vi "Run_FFID_Bkgnd.vi"(3 "Simulated Time":timestamp, 4 "Run Now?":bool, 5 "Simulate/Run":T3) -> (0 "Error Messages":string, 2 "Status":T1)   [LabVIEW 2018]
uses:
  Controls/User_Specific_mode.ctl
  Controls/Multirun_Execute_Row_Connector_Pane.ctl
  Gen Trav/Multi_Run_Status.ctl
  Globals/Trav_pos_global.vi
  Globals/Extra_Commands_Global.vi
  Globals/Constants_global.vi
panel:
  in  "User Specific":T2
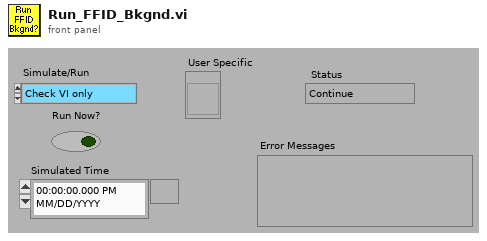
[diagram p1: front panel]
types:
  T1 = typedef "Multi_Run_Status.ctl" = enum16{"Continue", "Continue with Error", "Jump to Next Point", "Jump to Next Row", "Jump To Fall Back", "Terminate Run"}
  T2 = typedef "Multirun_Execute_Row_Connector_Pane.ctl" = refnum<vi>
  T3 = typedef "User_Specific_mode.ctl" = enum16{"Check VI only", "Run VI"}
  T4 = typedef "Traverse_cluster.ctl" = cluster{"Start X":sgl, "Start Y":sgl, "Start Z":sgl, "End X":sgl, "End Y":sgl, "End Z":sgl, "No. of pts.":i32, "Spacing":T5, "Filename":path, "Tunnel Speed":dbl, "Averaging time (min)":dbl, "Extra Commands":string, "Carrier_1 Q (l/min)":dbl, "Carrier_2 Q (l/min)":dbl, "Trace Gas Concentration (%)":dbl, "Specific Arguments":string, "Comments":string, "Row No":i32, "Row Type Selector":T6, "Completion time":string, "Row Duration (mins)":dbl, "No. of Valid pts.":i32, "Meas Setup File":string}
  T5 = typedef "Spacing.ctl" = enum16{"Linear", "Log", "Gauss", "Specified", "N/A"}
  T6 = typedef "Multi_run_mode.ctl" = enum16{"Move Traverse Only", "Set Tunnel Speed Only", "Set Source Only", "Set Measurement Conditions", "Single Measurement", "Vertical Profile", "Lateral Profile", "Longitudinal Profile", "Multi-Axis Profile", "Explore Volume", "Auto Calibrate", "Meas Fast FID Bkgnd", "Check Beam Power", "Scanning Valve Measurement", "Run VI Named:", "Set ADAM Ch", "Wait (minutes)", "Send Message", "Synchronize With:", "Fall Back to this Row", "Turn Off Row Repeating", "Traverse 3D Volume", "Blank Row", "Jump to Fall Back Row"}
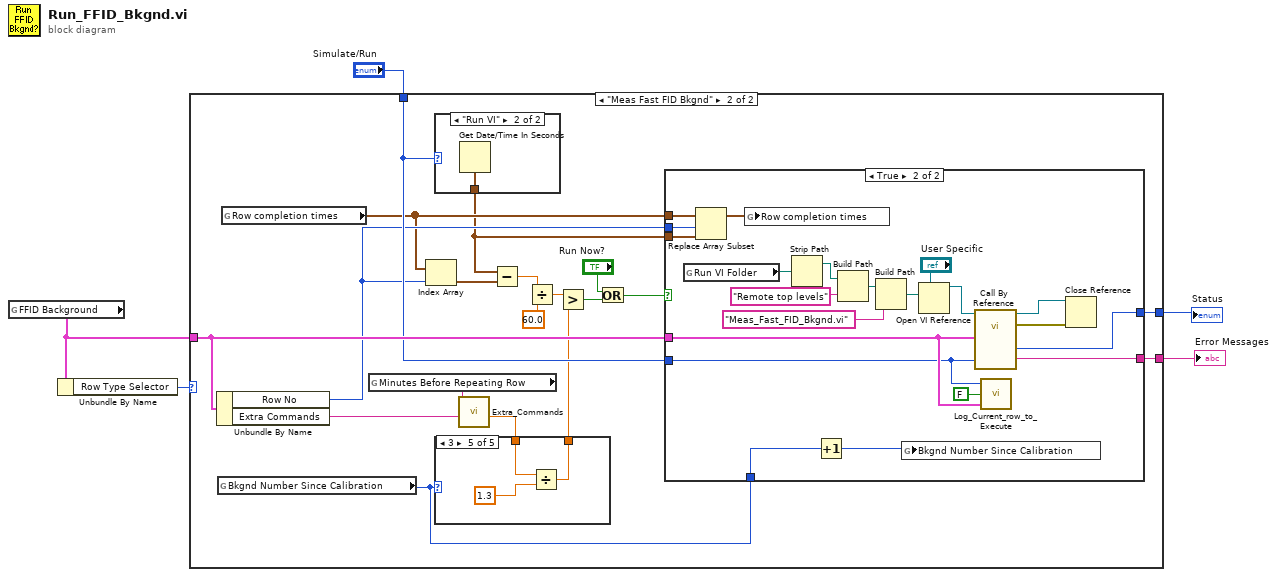
[diagram p0: block diagram]
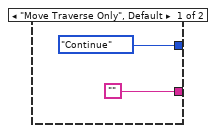
[diagram p2: hidden frame]
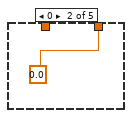
[diagram p4: hidden frame]
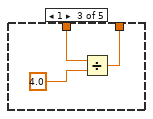
[diagram p5: hidden frame]
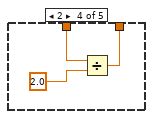
[diagram p6: hidden frame]
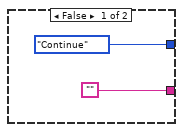
[diagram p7: hidden frame]
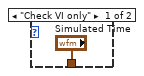
[diagram p8: hidden frame]
diagram:
  n1 = global read "Trav_pos_global.vi" "FFID Background"() -> (w5:T4)
  n2 = Unbundle By Name(w5) -> ("Row Type Selector"=w1:T6)
  n3 = case shown="\"Meas Fast FID Bkgnd\"" w1 {
    tunnel: w5 -> [_ w21]
    tunnel: "Simulate/Run" -> [_ w20]
    tunnel: [Multi_Run_Status."Continue" ("Status") w19] -> w3
    tunnel: ["" w18] -> w2
    frame "Move Traverse Only", Default {
    }
    frame "Meas Fast FID Bkgnd" {
      n4 = Unbundle By Name(w21) -> ("Row No"=w17:i32, "Extra Commands"=w11:string)
      n5 = global read "Trav_pos_global.vi" "Bkgnd Number Since Calibration"() -> (w8:i32)
      n6 = global read "Trav_pos_global.vi" "Row completion times"() -> (w16:timestamp[])
      n7 = global read "Extra_Commands_Global.vi" "Minutes Before Repeating Row"() -> (w26:string)
      n8 = Index Array(array=w16, index=w17) -> (element=w25:timestamp)
      n9 = case shown="\"Run VI\"" w20 {
        tunnel: ["Simulated Time" w62] -> w15
        frame "Check VI only" {
        }
        frame "Run VI" {
          n10 = Get Date/Time In Seconds() -> (seconds since 1Jan1904=w62:timestamp)
        }
      }
      n11 = call "Extra_Commands.vi"("String to Search"=w11, "Command"=w26) -> ("Numeric Value"=w9:dbl)  [unwired: 1 in, 4 out]
      n12 = case shown="3" w8 {
        tunnel: [w27 0.0 ("Numeric Value") w29 w32 w35] -> w10
        tunnel: w9 -> [w27 _ w31 w34 w37]
        frame Default {
        }
        frame 0 {
        }
        frame 1 {
          n13 = Divide(x=w31, y=4.0) -> (x/y=w29:dbl)
        }
        frame 2 {
          n14 = Divide(x=w34, y=2.0) -> (x/y=w32:dbl)
        }
        frame 3 {
          n15 = Divide(x=w37, y=1.3) -> (x/y=w35:dbl)
        }
      }
      n16 = Subtract(x=w15, y=w25) -> (x-y=w24:dbl)
      n17 = Divide(x=w24, y=60.0) -> (x/y=w23:dbl)
      n18 = Greater?(x=w23, y=w10) -> (0:w13:bool)
      n19 = Or(x="Run Now?", y=w13) -> (x .or. y?=w12:bool)
      n20 = case shown="True" w12 {
        tunnel: w21 -> [_ w43]
        tunnel: w20 -> [_ w42]
        tunnel: [Multi_Run_Status."Continue" ("Status") w50] -> w19
        tunnel: ["" w49] -> w18
        tunnel: w17 -> [_ w48]
        tunnel: w16 -> [_ w47]
        tunnel: w15 -> [_ w46]
        tunnel: w8 -> [_ w41]
        frame False {
        }
        frame True {
          n21 = global read "Constants_global.vi" "Run VI Folder"() -> (w60:path)
          n22 = Replace Array Subset(array=w47, new element=w46, index=w48) -> (w45:timestamp[])
          n23 = global write "Trav_pos_global.vi" "Row completion times"(w45) -> ()
          n24 = Strip Path(path=w60) -> (stripped path=w59:path)  [unwired: 1 out]
          n25 = Increment(x=w41) -> (x+1=w40:i32)
          n26 = Build Path(base path=w59, name or relative path="Remote top levels") -> (appended path=w56:path)
          n27 = Build Path(base path=w56, name or relative path="Meas_Fast_FID_Bkgnd.vi") -> (appended path=w52:path)
          n28 = global write "Trav_pos_global.vi" "Bkgnd Number Since Calibration"(w40) -> ()
          n29 = Open VI Reference(type specifier VI Refnum (for type only)="User Specific", vi path=w52) -> (vi reference=w51:T2)  [unwired: 2 in, 3 out]
          n30 = call-by-ref "?"(reference=w51, "Mode"=w42, "Traverse line In"=w43) -> (reference out=w54:T2, error out=w55:errorcluster, "Error Message"=w49:string, "Status"=w50:T1)  [unwired: 2 in, 1 out]
          n31 = call "Log_Current_row_to_Execute.vi"("Simulate/Run"=w42, "Start of Multi Run Prog"=FALSE, "Traverse line in"=w43) -> ()  [unwired: 2 in, 5 out]
          n32 = Close Reference(reference=w54, error in (no error)=w55) -> ()  [unwired: 1 out]
        }
      }
    }
  }
  "Status" <- w3
  "Error Messages" <- w2
